vi "Write to File.vi"(8 "error in":errorcluster, 11 "GUI Facade in":refnum<class "GUI Facade.lvclass">) -> (0 "error out":errorcluster, 3 "GUI Facade out":refnum<class "GUI Facade.lvclass">)   [LabVIEW 2015, in "GUI Facade.lvclass"]
uses:
  GUI Facade.lvclass
  GUI Facade.lvclass/GUI Facade.ctl
  File IO/Class/File Observer.lvclass
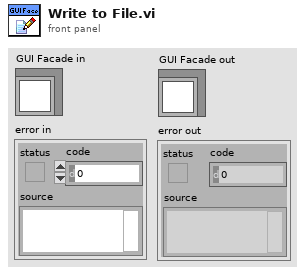
[diagram p1: front panel]
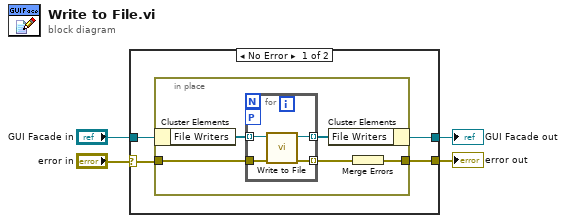
[diagram p0: block diagram]
diagram:
  n1 = case shown="No Error" "error in" {
    selector: "error in" -> [w7 w19]
    tunnel: [w6 w19] -> w3
    tunnel: [w5 w18] -> w1
    tunnel: "GUI Facade in" -> [w8 w18]
    frame No Error {
      n2 = in-place {
        in-place-border: w7 -> [w10]
        in-place-border: [w9] -> w6
        n3 = in-place-cluster #1(w8) -> ("File Writers"=w12:refnum<class "File Observer.lvclass">[])
        n4 = for {
          tunnel: w12 -> [w17] mode=indexing
          tunnel: [w16] -> w13 mode=indexing
          tunnel: [w15] -> w11 mode=indexing
          tunnel: w10 -> [w14]
          workers-P: _ -> [_]
          n5 = call "Write to File.vi"("error in"=w14, "File Obs in"=w17) -> ("error out"=w16:errorcluster, "File Obs out"=w15:refnum<class "File Observer.lvclass">)  [unwired: 8 in]
        }
        n6 = in-place-cluster #1("File Writers"=w11) -> (w5:refnum<class "GUI Facade.lvclass">)
        n7 = Merge Errors(w13) -> (w9:errorcluster)
      }
    }
    frame Error {
    }
  }
  "error out" <- w3
  "GUI Facade out" <- w1
